vi "8byte to 4 2byte.vi"(10 "payload":u8[](array[numeric])) -> (0 "7,6":i16, 1 "5,4":i16, 2 "3,2":i16, 3 "1,0":i16)   [LabVIEW 2014]
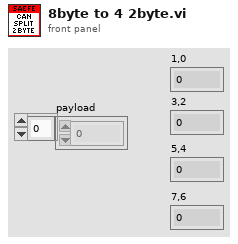
[diagram p1: front panel]
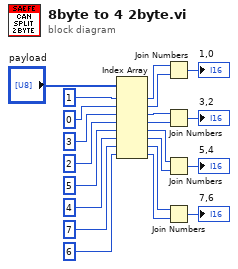
[diagram p0: block diagram]
diagram:
  n1 = Index Array(array="payload", index #1=1 ("index"), index #2=0 ("index"), index #3=3 ("index"), index #4=2 ("index"), index #5=5 ("index"), index #6=4 ("index"), index #7=7 ("index"), index #8=6 ("index")) -> (element #1=w14:u8, element #2=w15:u8, element #3=w16:u8, element #4=w17:u8, element #5=w18:u8, element #6=w19:u8, element #7=w20:u8, element #8=w21:u8)
  n2 = Join Numbers(hi=w14, lo=w15) -> ((hi.lo)=→"1,0":u16)
  n3 = Join Numbers(hi=w16, lo=w17) -> ((hi.lo)=→"3,2":u16)
  n4 = Join Numbers(hi=w18, lo=w19) -> ((hi.lo)=→"5,4":u16)
  n5 = Join Numbers(hi=w20, lo=w21) -> ((hi.lo)=→"7,6":u16)
